vi "Turn to Angle.vi"(0 "Current Angle (radians; 0 = right)":dbl, 1 "Target angle":dbl, 2 "Angle Tolerance":dbl=2.0, 3 "PID Gains":T1={"proportional gain (Kc)"=0.6, "integral time (Ti, min)"=0.0, "derivative time (Td, min)"=0.0} {"derivative time (Td, min)" format="%.3f"; "integral time (Ti, min)" format="%.3f"; "proportional gain (Kc)" format="%.3f"}, 4 "Max Output":dbl, 8 "reinitialize? (F)":bool) -> (5 "Turn Speed (subtact from the let motor output)":dbl, 7 "Finished?":bool)   [LabVIEW 2015]
uses:
  <vilib>/addons/control/pid/pid.llb/PID Control Input Filter (DBL).vi
  <vilib>/addons/control/pid/pid.llb/PID (DBL).vi
  <vilib>/addons/control/pid/NI_PID_pid.lvlib
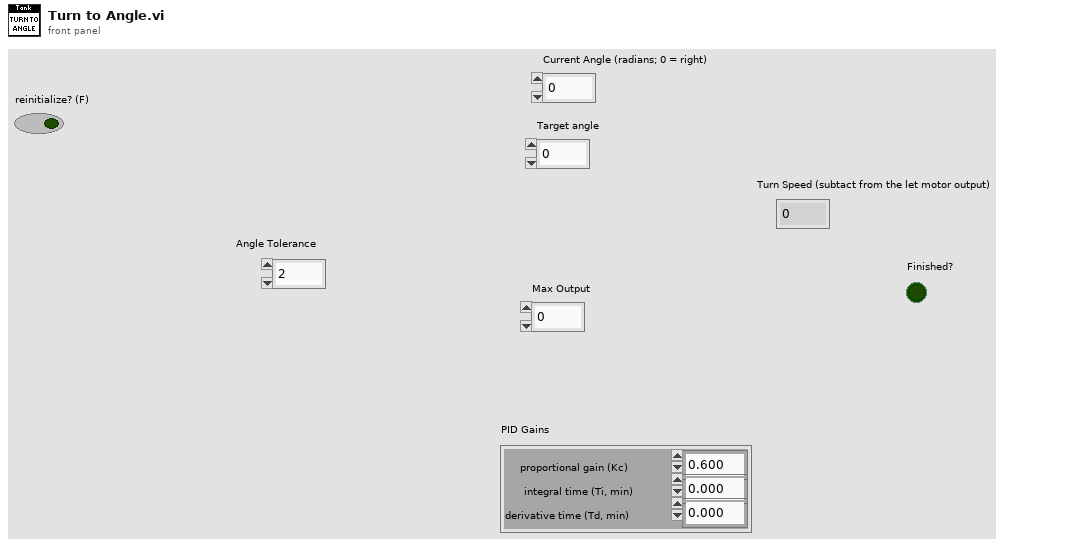
[diagram p1: front panel]
types:
  T1 = cluster{"proportional gain (Kc)":dbl, "integral time (Ti, min)":dbl, "derivative time (Td, min)":dbl}
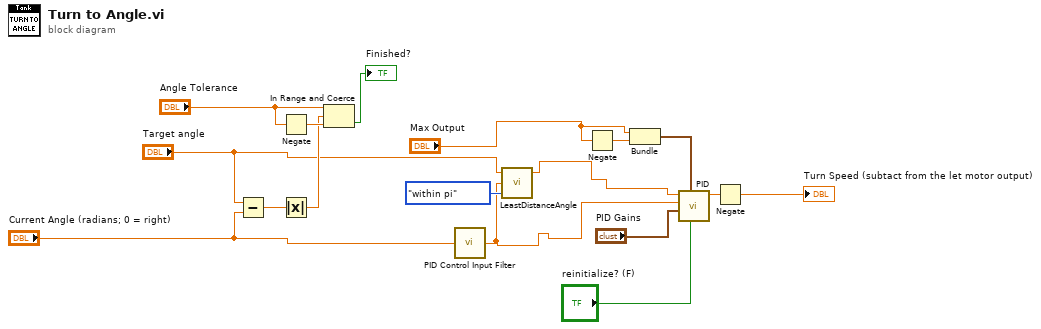
[diagram p0: block diagram]
diagram:
  n1 = Subtract(x="Target angle", y="Current Angle (radians; 0 = right)") -> (x-y=w16:dbl)
  n2 = Negate(x="Angle Tolerance") -> (-x=w14:dbl)
  n3 = Absolute Value(x=w16) -> (abs(x)=w12:dbl)
  n4 = In Range and Coerce(upper limit="Angle Tolerance", x=w12, lower limit=w14) -> (In Range?=→"Finished?":bool)  [unwired: 1 out]
  n5 = call-poly <vilib>:"PID Control Input Filter.vi"("input"="Current Angle (radians; 0 = right)") -> ("output"=w1:dbl)  [unwired: 4 in]
  n6 = call "LeastDistanceAngle.vi"("Enum"=enum16{"within pi", "within pi/2"}."within pi", "Current angle"=w1, "target angle (between pi and -pi) 2"="Target angle") -> ("output angle"=w2:dbl)  [unwired: 2 out]
  n7 = Negate(x="Max Output") -> (-x=w7:dbl)
  n8 = Bundle("Max Output"="Max Output", w7) -> (w6:cluster{"Max Output":dbl, dbl})  [unwired: 1 in]
  n9 = call-poly <vilib>:"PID.vi"("reinitialize? (F)"="reinitialize? (F)", "output range"=w6, "PID gains"="PID Gains", "process variable"=w1, "setpoint"=w2) -> ("output"=w9:dbl)  [unwired: 5 in, 1 out]
  n10 = Negate(x=w9) -> (-x=→"Turn Speed (subtact from the let motor output)":dbl)
